vi "PianoKeyboard.vi"(4 "起始音":T1={"音名"=enum."A", "度"=enum."0", "變音記號"=enum.""}, 6 "KeyNumbe":i32=12, 8 "error in (no error)":errorcluster) -> (0 "error out":errorcluster, 3 "Board":T2(plugin-control))   [LabVIEW 2015]
uses:
  Note.ctl
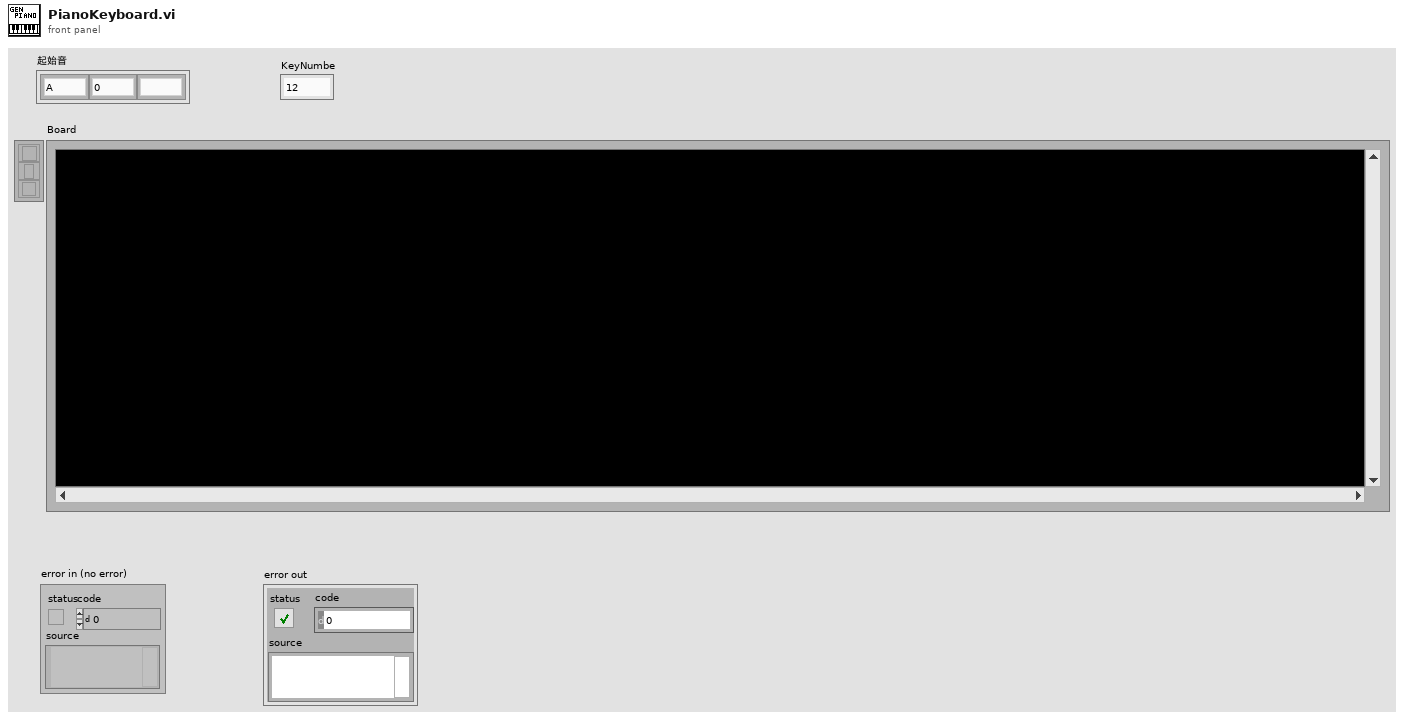
[diagram p1: front panel]
types:
  T1 = typedef "Note.ctl" = cluster{"音名":enum16{"C", "D", "E", "F", "G", "A", "B"}, "度":enum16{"0", "1", "2", "3", "4", "5", "6", "7", "8"}, "變音記號":enum16{"bb", "b", "", "#", "x"}}
  T2 = typedef "IMAQ Image.ctl" = refnum<image>
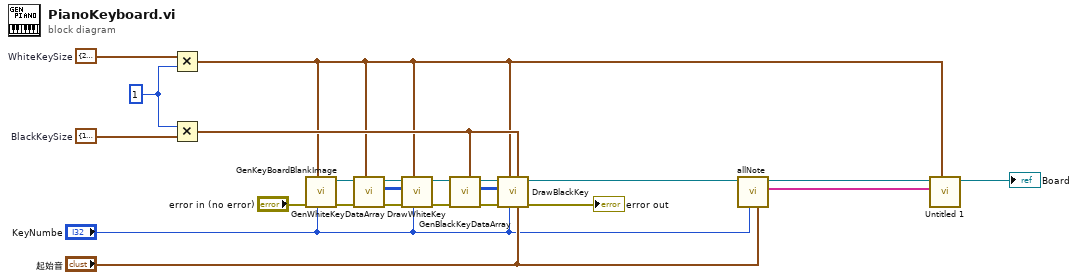
[diagram p0: block diagram]
diagram:
  w10 = 1
  w8 = cluster{"Width":i32, "Hieght":i32} {"Width"=10, "Hieght"=97}  # BlackKeySize
  w9 = cluster{"Width":i32, "Hieght":i32} {"Width"=21, "Hieght"=147}  # WhiteKeySize
  n1 = Multiply(x=w9, y=w10) -> (x*y=w1:cluster{"Width":i32, "Hieght":i32})
  n2 = Multiply(x=w10, y=w8) -> (x*y=w2:cluster{"Width":i32, "Hieght":i32})
  n3 = call "GenKeyBoardBlankImage.vi"("KeyNumber"="KeyNumbe", "WhiteKeySize"=w1, "error in (no error)"="error in (no error)") -> ("error out"=w13:errorcluster, "Image Out"=w14:T2)  [unwired: 7 in]
  n4 = call "GenWhiteKeyDataArray.vi"("WhiteKeySize"=w1, "error in (no error)"=w13) -> ("error out"=w19:errorcluster, "WhiteKeyData array"=w16:u32[][])  [unwired: 8 in]
  n5 = call "DrawWhiteKey.vi"("KeyNumber"="KeyNumbe", "WhiteKeySize"=w1, "error in (no error)"=w19, "WhiteKeyData array"=w16, "Image In"=w14) -> ("error out"=w18:errorcluster, "Image Out"=w20:T2)  [unwired: 5 in]
  n6 = call "GenBlackKeyDataArray.vi"("BlackKeySize"=w2, "error in (no error)"=w18) -> ("error out"=w17:errorcluster, "BlackKeyData array"=w15:u32[][])  [unwired: 8 in]
  n7 = call "DrawBlackKey.vi"("起始音"="起始音", "BlackKeySize"=w2, "KeyNumber"="KeyNumbe", "WhiteKeySize"=w1, "error in (no error)"=w17, "BlackKeyData array"=w15, "Image In"=w20) -> ("error out"=→"error out":errorcluster, "Image Out"=w3:T2)  [unwired: 3 in]
  n8 = call "allNote.vi"("起始音"="起始音", "KeyNumber"="KeyNumbe") -> ("音名Array"=w4:string[])  [unwired: 8 in, 1 out]
  n9 = call "Untitled 1.vi"("WhiteKeySize"=w1, "音名Array"=w4, "Image In"=w3) -> ("Image Out"=→"Board":T2)  [unwired: 7 in, 1 out]
